vi "PhaseSum9225-7_FPGA.vi"(3 "phi2 [pi rad]":fxp<+/-,36,2>, 5 "phi1 [pi rad]":fxp<+/-,36,2>) -> (1 "phi1+phi2 [pi rad] (-1,1]":fxp<+/-,36,2>)   [LabVIEW 2021]
uses:
  <vilib>/rvi/FXPMathLib/FxpAdd/XNode/nifxpmath_Add.xnode
  <vilib>/rvi/FXPMathLib/FxpInterpret/XNode/nifxpmath_Interpret.xnode
  <vilib>/rvi/FXPMathLib/FxpSub/XNode/nifxpmath_Sub.xnode
  <vilib>/rvi/FXPMathLib/sim/FxpSim.dll
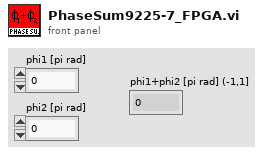
[diagram p1: front panel]
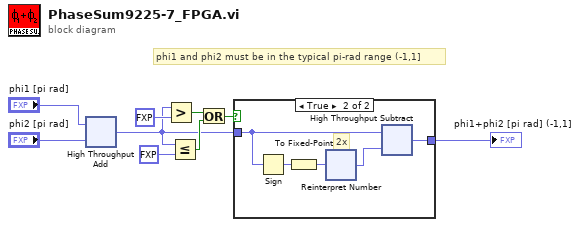
[diagram p0: block diagram]
diagram:
  # "phi1 and phi2 must be in the typical pi-rad range (-1,1]"
  n1 = xnode "High Throughput Add"("x"="phi1 [pi rad]", "y"="phi2 [pi rad]") -> ("x+y"=w1:fxp<+/-,36,2>)
  n2 = Greater?(x=w1, y=fxp<+,1,1> 1.0) -> (0:w7:bool)
  n3 = Less Or Equal?(x=w1, y=fxp<+/-,1,1> -1.0) -> (x <= y?=w6:bool)
  n4 = Or(x=w7, y=w6) -> (x .or. y?=w5:bool)
  n5 = case shown="True" w5 {
    tunnel: w1 -> [w10 w15]
    tunnel: [w10 w14] -> w4
    frame False {
    }
    frame True {
      # "2x"
      n6 = Sign(1:w15) -> (0:w12:fxp<+/-,2,2>)
      n7 = To Fixed-Point(number=w12) -> (fixed-point=w13:fxp<+/-,3,2>)  [unwired: 1 in]
      n8 = xnode "Reinterpret Number"("x"=w13) -> ("y"=w11:fxp<+/-,3,3>)
      n9 = xnode "High Throughput Subtract"("x"=w15, "y"=w11) -> ("x-y"=w14:fxp<+/-,36,2>)
    }
  }
  "phi1+phi2 [pi rad] (-1,1]" <- w4
